vi "Set Initialization Data - FPGA Read.vi"(8 "error in":errorcluster, 11 "cRIO NI 9205 Demo in":refnum<class "cRIO NI 9205 Demo.lvclass">) -> (0 "error out":errorcluster, 3 "cRIO NI 9205 Demo out":refnum<class "cRIO NI 9205 Demo.lvclass">)   [LabVIEW 2017, in "cRIO NI 9205 Demo.lvclass"]
doc: "In this VI you can set the initialization data of a statically-linked subWorker."
uses:
  cRIO NI 9205 Demo.lvclass
  FPGA Read/Initialization Data.ctl
  FPGA Read/Response Cases.ctl
  <vilib>/addons/_Workers/Library/Case Label.ctl
  cRIO NI 9205 Demo.lvclass/cRIO NI 9205 Demo.ctl
  FPGA Read/FPGA Read.lvclass
  C:/Program Files (x86)/National Instruments/LabVIEW 2017/vi.lib/addons/_Workers/Library/Classes/Worker/Worker.lvclass
  <vilib>/addons/_Workers/Library/Workers.lvlib
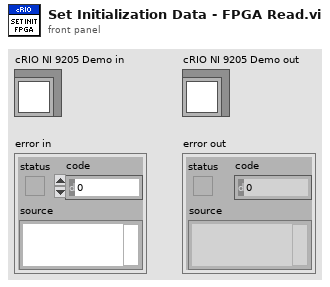
[diagram p1: front panel]
types:
  T1 = typedef "FPGA Read.lvclass/Initialization Data.ctl" = cluster{"Response Cases":T2}
  T2 = typedef "FPGA Read.lvclass/Response Cases.ctl" = cluster{"Receive FPGA Data":T3}
  T3 = typedef "Workers.lvlib/Case Label.ctl" = string
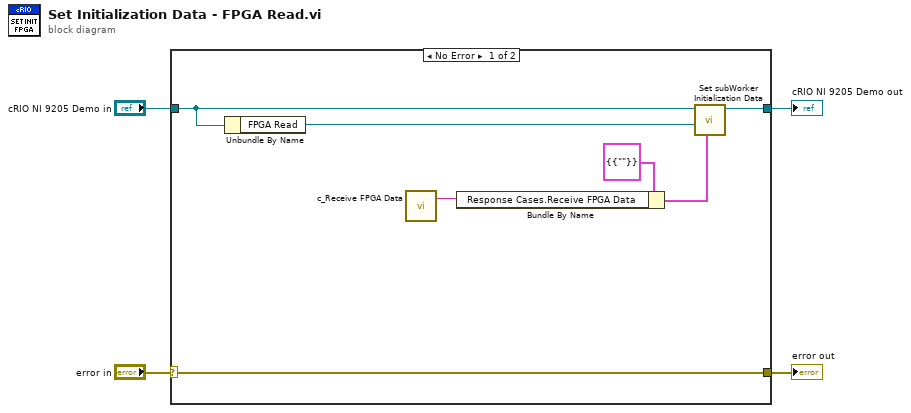
[diagram p0: block diagram]
diagram:
  n1 = case shown="No Error" "error in" {
    selector: "error in" -> [w11 w13]
    tunnel: [w11 w13] -> w3
    tunnel: [w9 w12] -> w2
    tunnel: "cRIO NI 9205 Demo in" -> [w6 w12]
    frame No Error {
      n2 = Unbundle By Name(w6) -> ("FPGA Read"=w10:refnum<class "FPGA Read.lvclass">)
      n3 = call "c_Receive FPGA Data.vi"() -> ("Case Label"=w5:T3)  [unwired: 1 in]
      n4 = Bundle By Name(cluster=T1 {"Response Cases"={"Receive FPGA Data"=""}} ("Initialization Data"), "Response Cases.Receive FPGA Data"=w5) -> (w7:T1)
      n5 = call-dynamic "Set subWorker Initialization Data.vi"("Initialization Data"=w7, "subWorker"=w10, "Worker"=w6) -> ("Worker out"=w9:refnum<class "cRIO NI 9205 Demo.lvclass">)  [unwired: 8 in]
    }
    frame Error {
    }
  }
  "error out" <- w3
  "cRIO NI 9205 Demo out" <- w2
